vi "TSP_GA.vi"(5 "Number of Iterative":dbl, 7 "pop_size":dbl, 8 "error in":errorcluster, 9 "Pop in":dbl[][](array[numeric]), 11 "xy":dbl[][](array[numeric])) -> (0 "error out":errorcluster, 1 "pop out":dbl[][](array[numeric]), 2 "min dist":dbl, 3 "opt_rte":i16[](array[numeric]), 4 "Time Cost":u32)   [LabVIEW 2016]
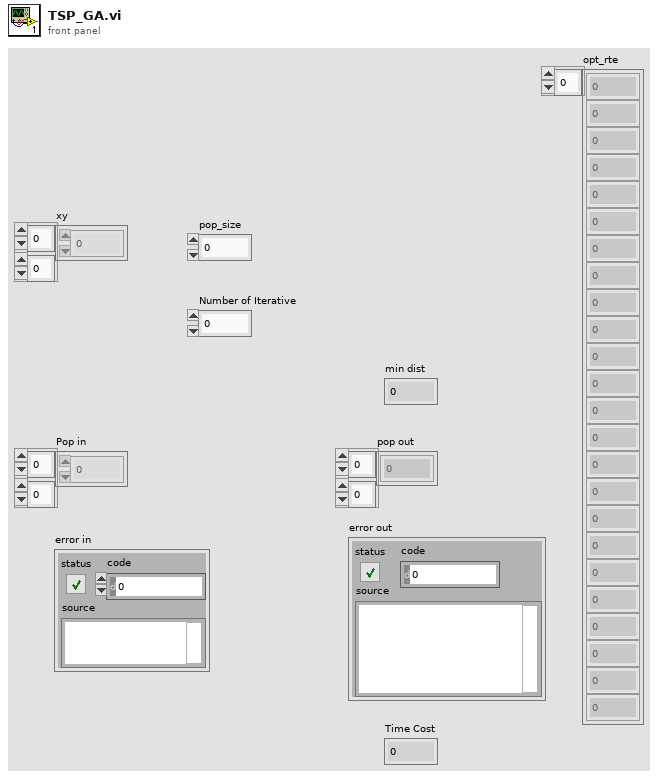
[diagram p1: front panel]
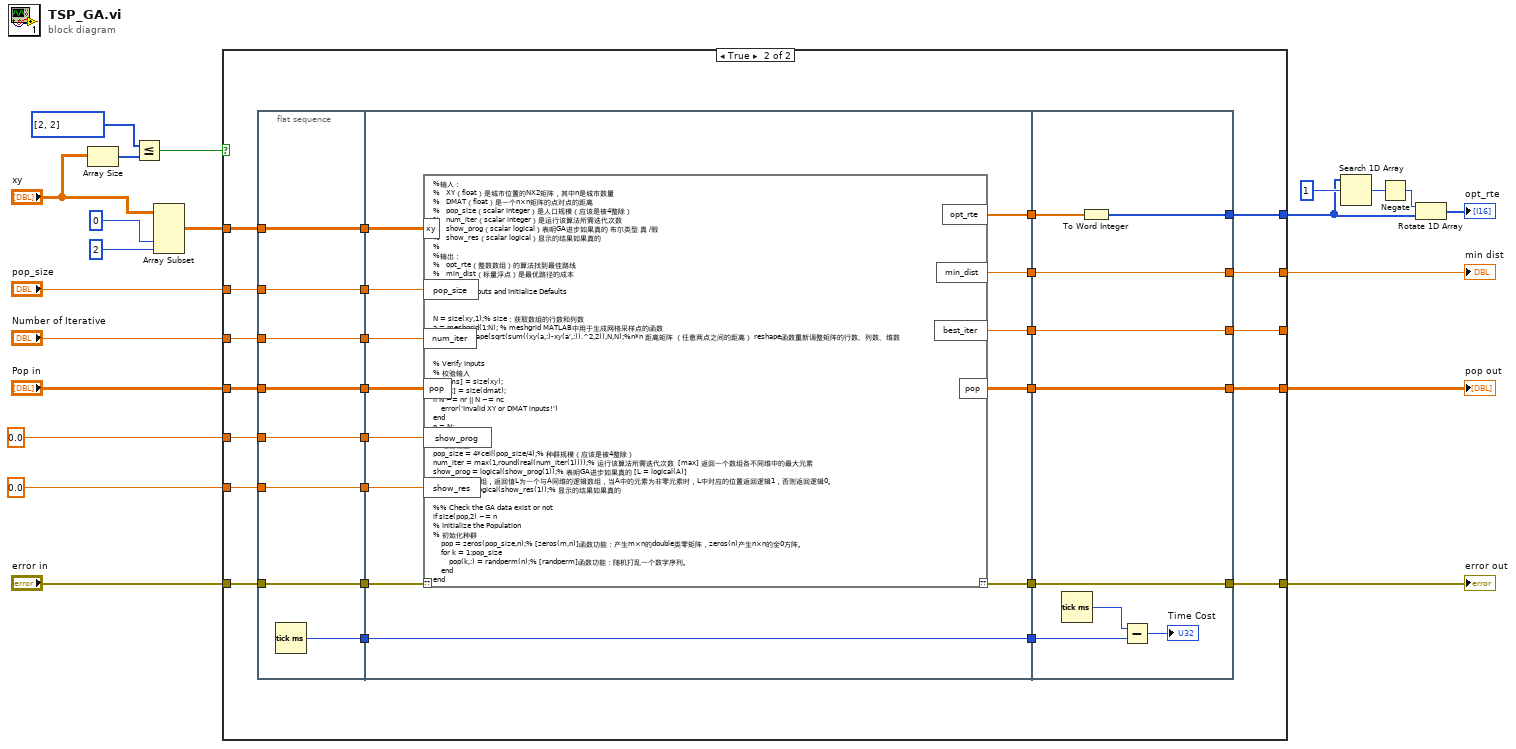
[diagram p0: block diagram]
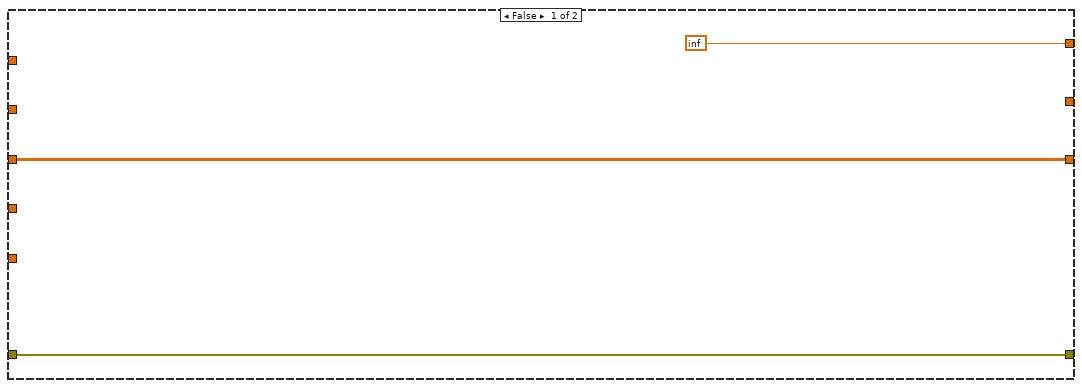
[diagram p2: hidden frame]
diagram:
  n1 = Array Size(array="xy") -> (size(s)=w21:i32[])
  n2 = Less Or Equal?(x=i32[] [2, 2] ("y"), y=w21) -> (x <= y?=w19:bool)
  n3 = Array Subset(array="xy", index (col)=0 ("index"), length (col)=2 ("length")) -> (w16:dbl[][])  [unwired: 2 in]
  n4 = case shown="True" w19 {
    tunnel: w16 -> [_ w47]
    tunnel: "pop_size" -> [_ w45]
    tunnel: "Number of Iterative" -> [_ w43]
    tunnel: "Pop in" -> [w23 w41]
    tunnel: 0.0 ("Real") -> [_ w39]
    tunnel: 0.0 ("Real") -> [_ w37]
    tunnel: "error in" -> [w22 w35]
    tunnel: [_ w34] -> w2
    tunnel: [inf w33] -> w5
    tunnel: [_ w31] -> _
    tunnel: [w23 w29] -> w4
    tunnel: [w22 w27] -> w3
    frame False {
    }
    frame True {
      n5 = flat-sequence {
        tunnel: [w58] -> w50
        tunnel: [w57] -> w48
        tunnel: w47 -> [w57]
        tunnel: [w56] -> w46
        tunnel: w45 -> [w56]
        tunnel: [w55] -> w44
        tunnel: w43 -> [w55]
        tunnel: [w54] -> w42
        tunnel: w41 -> [w54]
        tunnel: [w53] -> w40
        tunnel: w39 -> [w53]
        tunnel: [w52] -> w38
        tunnel: w37 -> [w52]
        tunnel: [w51] -> w36
        tunnel: w35 -> [w51]
        tunnel: w50 -> [w71]
        tunnel: [w71] -> w49
        tunnel: w48 -> [w70]
        tunnel: w46 -> [w69]
        tunnel: w44 -> [w68]
        tunnel: w42 -> [w67]
        tunnel: w40 -> [w66]
        tunnel: w38 -> [w65]
        tunnel: w36 -> [w64]
        tunnel: [w63] -> w32
        tunnel: [w62] -> w30
        tunnel: [w61] -> w28
        tunnel: [w60] -> w26
        tunnel: [w59] -> w25
        tunnel: w49 -> [w79]
        tunnel: [w73] -> w34
        tunnel: [w77] -> w33
        tunnel: w32 -> [w77]
        tunnel: [w76] -> w31
        tunnel: w30 -> [w76]
        tunnel: [w75] -> w29
        tunnel: w28 -> [w75]
        tunnel: [w74] -> w27
        tunnel: w26 -> [w74]
        tunnel: w25 -> [w72]
        frame #0 {
          n6 = Tick Count (ms)() -> (millisecond timer value=w58:u32)
        }
        frame #1 {
          n7 = script code="%输入：\n%   XY（float）是城市位置的NX2矩阵，其中n是城市数量\n%   DMAT（float）是一个n×n矩阵的点对点的距离\n%   pop_size（scalar integer）是人口规模（应该是被4整除）\n%   num_iter（scalar integer）是运行该算法所需迭代次数\n%   show_prog（scalar logical）表明GA进步如果真的 布尔类型 真 /假\n%   show_res（scalar logical）显示的结果如果真的\n%\n%输出：\n%   opt_rte（整数数组）的算法找到最佳路线\n%   min_dist（标量浮点）是最优路径的成本\n\n% Process Inputs and Initialize Defaults  \n\n\nN = size(xy,1);% size：获取数组的行数和列数\na = meshgrid(1:N); % meshgrid MATLAB中用于生成网格采样点的函数\ndmat = reshape(sqrt(sum((xy(a,:)-xy(a',:)).^2,2)),N,N);%n*n 距离矩阵 （任意两点之间的距离） reshape函数重新调整矩阵的行数、列数、维数\n\n\n% Verify Inputs\n% 校验输入\n[N,dims] = size(xy);\n[nr,nc] = size(dmat);\nif N ~= nr || N ~= nc\n    error('Invalid XY or DMAT inputs!')\nend\nn = N;\n% Sanity Checks\n% 理智检查\npop_size = 4*ceil(pop_size/4);% 种群规模（应该是被4整除）\nnum_iter = max(1,round(real(num_iter(1))));% 运行该算法所需迭代次数  [max] 返回一个数组各不同维中的最大元素\nshow_prog = logical(show_prog(1));% 表明GA进步如果真的 [L = logical(A)] 输入A为实数数组，返回值L为一个与A同维的逻辑数组，当A中的元素为非零元素时，L中对应的位置返回逻辑1，否则返回逻辑0。\nshow_res = logical(show_res(1));% 显示的结果如果真的\n\n%% Check the GA data exist or not\nif size(pop,2) ~= n\n% Initialize the Population\n% 初始化种群\n    pop = zeros(pop_size,n);% [zeros(m,n)]函数功能：产生m×n的double类零矩阵，zeros(n)产生n×n的全0方阵。\n    for k = 1:pop_size\n        pop(k,:) = randperm(n);% [randperm]函数功能：随机打乱一个数字序列。\n    end\nend\n\n\n%% Run the GA\n% 运行遗传算法\nopt_rte = []; % 最佳路径\nrte = []; % 最佳路径 回环\nglobal_min = Inf;% 最优路径的距离\ntotal_dist = zeros(1,pop_size);% 总距离矩阵 1*种群大小\nmin_dist = Inf ; % 最优路径的总距离\ndist_history = zeros(1,num_iter);% 生成1*代数维的零矩阵\ntmp_pop = zeros(4,n);% 缓存种群4*n 维的零矩阵\nnew_pop = zeros(pop_size,n);% 新种群 种群大小*n维的零矩阵\nif show_prog% 当进化有效\n    %pfig = figure('Name','TSP_GA | Current Best Solution');%绘图\nend\nbest_iter = num_iter ; \nfor iter = 1:num_iter\n    % Evaluate Each Population Member (Calculate Total Distance)\n    % 任意两个城市之间的距离和（并计算总距离 d）\n    for p = 1:pop_size\n        d = dmat(pop(p,n),pop(p,1)); % Closed Path 封闭路径\n        for k = 2:n\n            d = d + dmat(pop(p,k-1),pop(p,k));\n        end\n        total_dist(p) = d;% 任意两个城市之间的距离和的和\n    end\n    % Find the Best Route in the Population\n    % 在种群中找到最佳路线 \n    [min_dist,index] = min(total_dist);% [min()]返回一个数组各不同维中的最小元素\n    dist_history(iter) = min_dist;\n    if min_dist < global_min% 保留距离最小值\n        global_min = min_dist;\n        opt_rte = pop(index,:);\n        best_iter = iter;\n        rte = opt_rte([1:n 1]);\n        if show_prog\n            % Plot the Best Route\n            % 绘制最佳路线\n            figure(1);% figure 能够创建一个用来显示图形输出的一个窗口对象\n            \n            if dims == 3, plot3(xy(rte,1),xy(rte,2),xy(rte,3),'r.-');% 创建一个三维坐标下的图\n            else plot(xy(rte,1),xy(rte,2),'r.-'); end\n            title(sprintf('Total Distance = %1.4f, Iteration = %d',min_dist,iter));\n        end\n    end\n    % Genetic Algorithm Operators\n    % 遗传算法\n    rand_pair = randperm(pop_size);% randperm 函数功能：随机打乱一个数字序列。\n    for p = 4:4:pop_size\n        rtes = pop(rand_pair(p-3:p),:);     % my 每四个排序方式组成一组\n        dists = total_dist(rand_pair(p-3:p));  % my 取出这四个排序方式的总路程\n        [ignore,idx] = min(dists); % my 四个排序中的最短路程\n        best_of_4_rte = rtes(idx,:); \n        ins_pts = sort(ceil(n*rand(1,2)));% [sort(A)]若A是向量不管是列还是行向量，默认都是对A进行升序排列 [ceil(n)]的意思是向正方向舍入\n                                          % my 随机选出两个城市 （升序）\n        I = ins_pts(1);% 取出两个维度的坐标\n        J = ins_pts(2);\n        % 变异\n        for k = 1:4 % Mutate the Best to get Three New Routes 变异最好得到第三条路线\n            tmp_pop(k,:) = best_of_4_rte;  % my 对这一组4个方案中的最佳方案进行进化\n            switch k\n                case 2 % Flip 翻转\n                    tmp_pop(k,I:J) = fliplr(tmp_pop(k,I:J));  % my 取任意一段反转\n                case 3 % Swap 交换\n                    tmp_pop(k,[I J]) = tmp_pop(k,[J I]);    % my 交换任意两个城市的顺序\n                case 4 % Slide 循环移位\n                    tmp_pop(k,I:J) = tmp_pop(k,[I+1:J I]);  % my 任意一段 循环移位\n                otherwise % Do Nothing\n            end\n        end\n        new_pop(p-3:p,:) = tmp_pop;\n    end\n    pop = new_pop;\nend\n\n\nif show_res\n    %Plots the GA Results\n    %绘制遗传算法结果\n    figure(2);\n    \n    % 城市位置\n    subplot(2,2,1);\n    if dims == 3, plot3(xy(:,1),xy(:,2),xy(:,3),'k.');\n    else plot(xy(:,1),xy(:,2),'k.'); end\n    title('City Locations');\n    \n    % 距离矩阵\n    subplot(2,2,2);\n    imagesc(dmat(opt_rte,opt_rte));\n    title('Distance Matrix');\n    \n    % 总距离\n    subplot(2,2,3);\n    rte = opt_rte([1:n 1]);\n    if dims == 3, plot3(xy(rte,1),xy(rte,2),xy(rte,3));% plot3(x,y,z)用来绘制3维曲线图\n    else plot(xy(rte,1),xy(rte,2)); end\n    title(sprintf('Total Distance = %1.4f',min_dist));\n    \n    % 最佳\n    subplot(2,2,4);\n    plot(dist_history,'b','LineWidth',2);\n    title('Best Solution History');\n    set(gca,'XLim',[0 num_iter+1],'YLim',[0 1.1*max([1 dist_history])]); %[set] Matlab中“坐标轴刻度”的不同风格 \nend\n\n%% Return Outputs\n% 返回结果"("??"=w64, "xy"=w70, "pop_size"=w69, "num_iter"=w68, "pop"=w67, "show_prog"=w66, "show_res"=w65) -> ("??"=w60:errorcluster, "opt_rte"=w59:dbl[], "min_dist"=w63:dbl, "best_iter"=w62:dbl, "pop"=w61:dbl[][])
        }
        frame #2 {
          n8 = Tick Count (ms)() -> (millisecond timer value=w80:u32)
          n9 = To Word Integer(number=w72) -> (16bit integer=w73:i16[])
          n10 = Subtract(x=w80, y=w79) -> (x-y=→"Time Cost":u32)
        }
      }
    }
  }
  "pop out" <- w4
  "min dist" <- w5
  "error out" <- w3
  n11 = Search 1D Array(1D array=w2, element=i16 1) -> (index of element=w7:i32)  [unwired: 1 in]
  n12 = Negate(x=w7) -> (-x=w8:i32)
  n13 = Rotate 1D Array(1:w2, 2:w8) -> (0:→"opt_rte":i16[])
